vi "Add Data Replay Offset RTM.vi"(8 "error in (no error)":errorcluster, 11 "Node Ptr":u64 format="%.0x") -> (0 "error out":errorcluster)   [LabVIEW 2011, in "Engine Sim System Explorer.lvlib"]
uses:
  Engine Sim System Explorer.lvlib
  <vilib>/NI Veristand/Custom Device API/Custom Device Channel.ctl
  <vilib>/NI Veristand/Custom Device API/Custom Device Channel Type.ctl
  Shared/Engine Simulation Global.vi
  <vilib>/NI Veristand/Custom Device API/Custom Device API.lvlib
  <vilib>/NI Veristand/Custom Device Tools/Custom Device Utility Library/Custom Device Utility Library.lvlib
  Engine Simulation Shared.lvlib
panel:
  in  "Tag":string
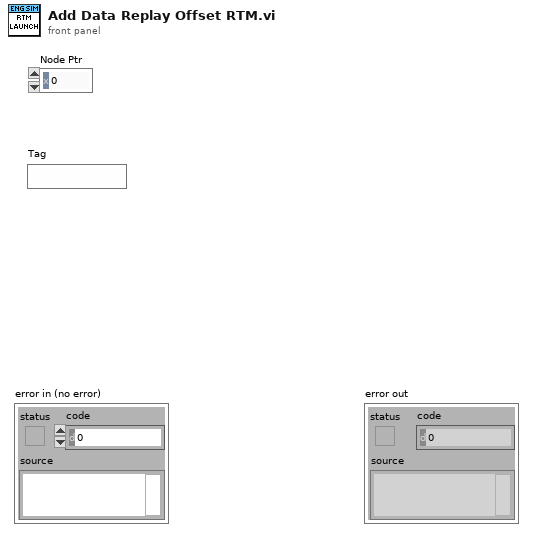
[diagram p1: front panel]
types:
  T1 = typedef "Custom Device API.lvlib/Custom Device Channel.ctl" = cluster{"Type":T2, "Units":string, "Default Value":dbl, "Faultable":bool, "Scalable":bool}
  T2 = typedef "Custom Device API.lvlib/Custom Device Channel Type.ctl" = enum16{"Input", "Output"}
  T3 = typedef "Custom Device API.lvlib/Custom Device Item Ref.ctl" = u64
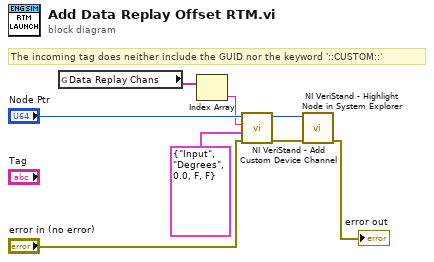
[diagram p0: block diagram]
diagram:
  # "The incoming tag does neither include the GUID nor the keyword '::CUSTOM::'"
  n1 = global read "Engine Simulation Global.vi" "Data Replay Chans"() -> (w2:string[])
  n2 = Index Array(array=w2) -> (element=w1:string)  [unwired: 1 in]
  n3 = call <vilib>:"NI VeriStand - Add Custom Device Channel.vi"("error in (no error)"="error in (no error)", "Channel"=T1 {"Type"=enum."Input", "Units"="Degrees", "Default Value"=0.0, "Faultable"=FALSE, "Scalable"=FALSE}, "Channel Name"=w1, "Parent Ref in"="Node Ptr") -> ("error out"=w5:errorcluster, "Parent Ref out"=w4:T3)  [unwired: 4 in, 2 out]
  n4 = call <vilib>:"NI VeriStand - Highlight Node in System Explorer.vi"("error in (no error)"=w5, "Item Ref in"=w4) -> ("error out"=→"error out":errorcluster)  [unwired: 8 in, 1 out]
